vi "Set Server Address.vi"(10 "Server Address":string, 11 "OOP Server in":refnum<class "helloWServer.lvclass">) -> (3 "OOP Server out":refnum<class "helloWServer.lvclass">)   [LabVIEW 2020, in "helloWServer.lvlib" / "helloWServer.lvclass"]
uses:
  helloWServer.lvclass
  helloWServer.lvclass/helloWServer.ctl
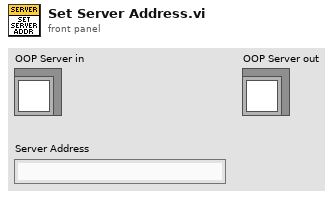
[diagram p1: front panel]
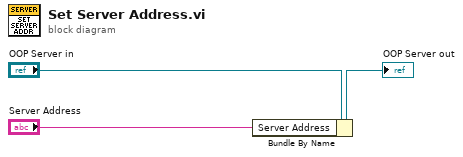
[diagram p0: block diagram]
diagram:
  n1 = Bundle By Name(cluster="OOP Server in", "Server Address"="Server Address") -> (→"OOP Server out":refnum<class "helloWServer.lvclass">)
